vi "5 ch 2 samples minimum resonance scanner (FPGA) fixed pix clock.vi"() -> ()   [LabVIEW 2012]
uses:
  <vilib>/eio/EIONode/EIONode.xnode
  <vilib>/rvi/eio/common/nirviEmuTemplateMethod_errors.vi
  <vilib>/rvi/DataTransferAndStorage/Container/XNode/niFpgaContainer.xnode
  <vilib>/platform/TimedLoop/XDataNode/XDataNode.xnode
  <vilib>/Platform/TimedLoop/XDataNode/nitl_modes.ctl
  <vilib>/Platform/TimedLoop/XDataNode/XDNodeRunTimeDep.lvlib
  <vilib>/Platform/TimedLoop/XDataNode/wakeup.ctl
  <vilib>/Platform/TimedLoop/XDataNode/timing_clust.ctl
  <vilib>/rvi/interface/RandomDataEmulation/nirviRandomDataFpgaReadWriteTemplate.vi
panel:
  in  "lines at once":i16=4999
  in  "samples per half period":i16=4999
  in  "Start Delay (Ticks)":i16 caption="Start delay (Ticks)"
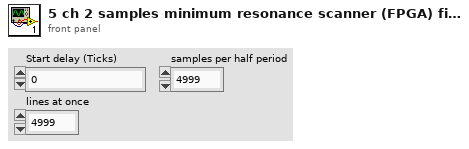
[diagram p1: front panel]
types:
  T1 = cluster{"IO Module\\AI A0":i16, "IO Module\\AI A1":i16, "IO Module\\AI A3":i16, "IO Module\\AI A6":i16}
  T2 = typedef "XDNodeRunTimeDep.lvlib/timing_clust.ctl" = cluster{"Expected End [f-1]":u64, "Actual End [f-1]":u64, "Finished Late? [f-1]":bool, "Expected End [i-1]":u64, "Actual End [i-1]":u64, "Finished Late? [i-1]":bool, "Expected Start [i]":u64, "Actual Start [i]":u64, "Expected Start [f]":u64, "Actual Start [f]":u64, "Source Name":string, "Structure Name":string, "Period":i64, "Deadline":i64, "Offset":i64, "Start":i64, "Priority":i32, "Timeout":i32, "Mode":T3, "Wakeup Reason":T4, "Error":errorcluster, "Source Type":string, "Secondary Source Type":string, "Global End Time":u64, "Global Start Time":u64, "Frame Duration":u64, "Iteration Duration":u64, "Assigned CPU":i32, "I/O Scan Engine Mode":u32}
  T3 = typedef "XDNodeRunTimeDep.lvlib/nitl_modes.ctl" = enum32{"No Change", "Process missed periods, maintain original phase", "Discard missed periods, maintain original phase", "Process missed periods, ignore original phase", "Discard missed periods, ignore original phase"}
  T4 = typedef "XDNodeRunTimeDep.lvlib/wakeup.ctl" = enum32{"Normal", "Aborted", "Asynchronous wakeup", "Timing source error", "Timed loop error", "Timeout"}
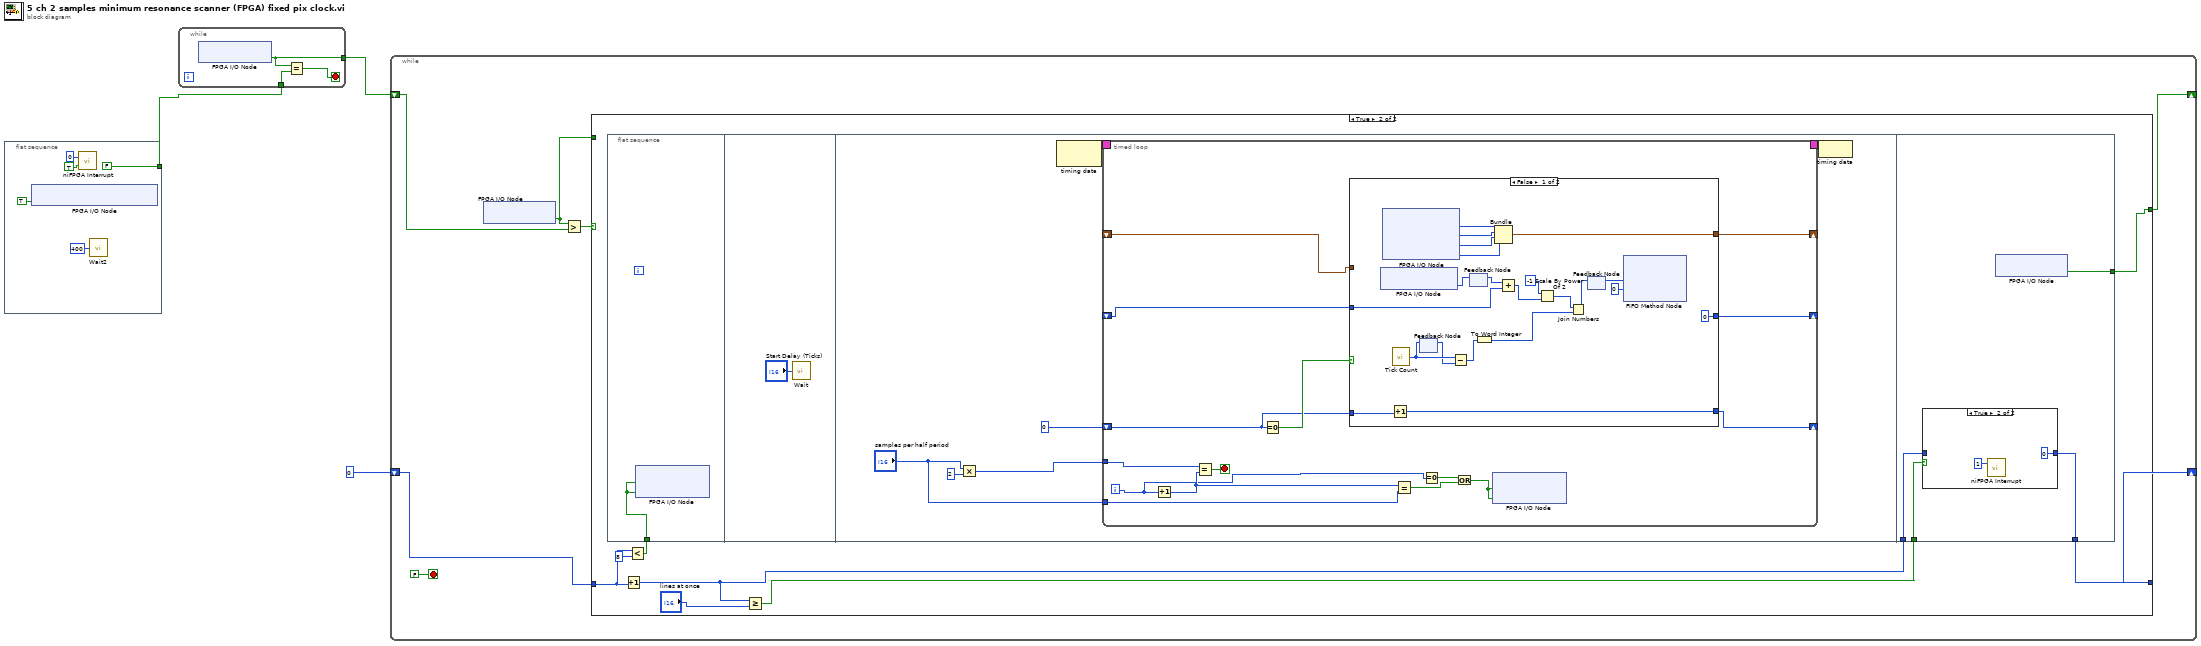
[diagram p0: block diagram]
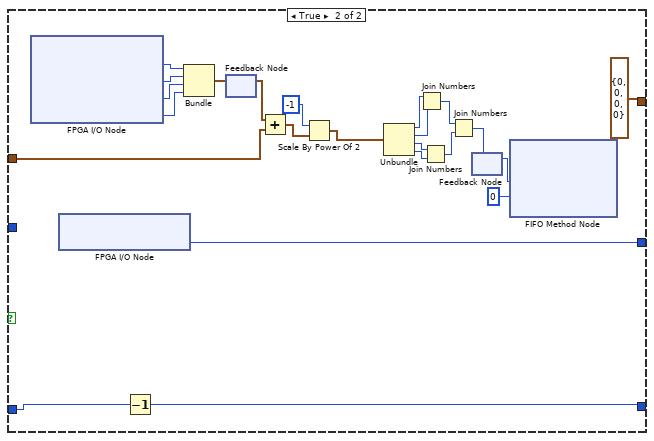
[diagram p3: hidden frame]
diagram:
  n1 = flat-sequence {
    tunnel: [FALSE ("IO Module\\DI 0")] -> w2
    frame #0 {
      n2 = xnode "FPGA I/O Node"("IO Module\\Digital Output Enable"=TRUE ("IO Module\\Digital Output Enable")) -> ()  [unwired: 1 in, 1 out]
      n3 = call <vilib>:"niFPGA Interrupt.vi"("Wait Until Cleared (F)"=TRUE, "IRQ Number (0)"=u8 0) -> ()  [unwired: 1 in]
      n4 = call "Wait2"("Count(mSec)"=u32 400) -> ()  [unwired: 1 out]
    }
  }
  n5 = while {
    tunnel: w2 -> [w11]
    tunnel: [w9] -> w1
    stop <- w10 stop-if-true
    n6 = xnode "FPGA I/O Node"() -> ("IO Module\\DI 0"=w9:bool)  [unwired: 1 in, 1 out]
    n7 = Equal?(x=w9, y=w11) -> (x = y?=w10:bool)
  }
  n8 = while {
    shift-right: [w17] -> _
    shift-left: w1 -> [w18]
    shift-right: [w15] -> _
    shift-left: i16 0 ("IRQ Number (0)") -> [w14]
    stop <- FALSE stop-if-true
    n9 = xnode "FPGA I/O Node"() -> ("IO Module\\DI 0"=w12:bool)  [unwired: 1 in, 1 out]
    n10 = Greater?(x=w12, y=w18) -> (0:w13:bool)
    n11 = case shown="True" w13 {
      tunnel: [w19 w21] -> w17
      tunnel: w14 -> [w20 w24]
      tunnel: [w20 w26] -> w15
      tunnel: w12 -> [w19 _]
      frame False {
      }
      frame True {
        n12 = flat-sequence {
          tunnel: w22 -> [w29]
          tunnel: w28 -> [w103]
          tunnel: w27 -> [w102]
          tunnel: [w101] -> w26
          tunnel: [w100] -> w21
          frame #0 {
            n13 = xnode "FPGA I/O Node"("PXI_Trig2"=w29, "IO Module\\D0 2"=w29) -> ()  [unwired: 2 in, 2 out]
          }
          frame #1 {
            n14 = call "Wait"("Count(Ticks)"="Start Delay (Ticks)") -> ()  [unwired: 1 out]
          }
          frame #2 {
            n15 = Multiply(x="samples per half period", y=i16 2) -> (x*y=w35:i16)
            n16 = node-c288() -> (w34:T2)  [unwired: 1 in]
            n17 = timed-loop {
              tunnel: w35 -> [w50]
              timing: w34 -> [_]
              timing-out: [_] -> w33
              shift-right: [w47] -> _
              shift-left: 0 ("Timeout") -> [w48]
              tunnel: "samples per half period" -> [w42]
              shift-right: [w40] -> _
              shift-left: _ -> [w39]
              shift-right: [w38] -> _
              shift-left: _ -> [w37]
              i -> [w41]
              stop <- w51 stop-if-true
              n18 = Increment(x=w41) -> (x+1=w43:i32)
              n19 = Equal?(x=w50, y=w43) -> (x = y?=w51:bool)
              n20 = Equal To 0?(x=w48) -> (x = 0?=w49:bool)
              n21 = case shown="False" w49 {
                tunnel: w48 -> [w72 w94]
                tunnel: [w71 w93] -> w47
                tunnel: [w61 T1 {"IO Module\\AI A0"=0, "IO Module\\AI A1"=0, "IO Module\\AI A3"=0, "IO Module\\AI A6"=0}] -> w40
                tunnel: w39 -> [_ w84]
                tunnel: [i16 0 ("IO Module\\AI B8") w77] -> w38
                tunnel: w37 -> [w58 _]
                frame False {
                  n22 = xnode "FPGA I/O Node"() -> ("IO Module\\AI B8"=w60:i16)  [unwired: 1 in, 1 out]
                  n23 = xnode "FPGA I/O Node"() -> ("IO Module\\AI A0"=w65:i16, "IO Module\\AI A1"=w64:i16, "IO Module\\AI A3"=w63:i16, "IO Module\\AI A6"=w62:i16)  [unwired: 4 in, 4 out]
                  n24 = Increment(x=w72) -> (x+1=w71:i32)
                  n25 = call "Tick Count"() -> ("Tick Count(Ticks)"=w70:u32)
                  n26 = feedback #1() -> (w69:u32)  [unwired: 1 in]
                  n27 = feedback-in #1(w70) -> ()
                  n28 = Subtract(x=w70, y=w69) -> (x-y=w68:u32)
                  n29 = feedback-in #2(w60) -> ()
                  n30 = feedback #2() -> (w59:i16)  [unwired: 1 in]
                  n31 = To Word Integer(number=w68) -> (16bit integer=w66:i16)
                  n32 = Bundle("IO Module\\AI A0"=w65, "IO Module\\AI A1"=w64, "IO Module\\AI A3"=w63, "IO Module\\AI A6"=w62) -> (w61:T1)  [unwired: 1 in]
                  n33 = Add(x=w59, y=w58) -> (x+y=w54:i16)
                  n34 = Scale By Power Of 2(n=i16 -1, x=w54) -> (x*2^n=w53:i16)
                  n35 = Join Numbers(hi=w53, lo=w66) -> ((hi.lo)=w57:u32)
                  n36 = feedback-in #3(w57) -> ()
                  n37 = feedback #3() -> (w52:u32)  [unwired: 1 in]
                  n38 = xnode ("FIFO Method Node")("Element"=w52, "Timeout"=0) -> ()  [unwired: 1 in, 2 out]
                }
                frame True {
                  n39 = xnode "FPGA I/O Node"() -> ("IO Module\\AI A0"=w90:i16, "IO Module\\AI A1"=w89:i16, "IO Module\\AI A3"=w88:i16, "IO Module\\AI A6"=w87:i16)  [unwired: 4 in, 4 out]
                  n40 = xnode "FPGA I/O Node"() -> ("IO Module\\AI B8"=w77:i16)  [unwired: 1 in, 1 out]
                  n41 = Decrement(x=w94) -> (x-1=w93:i32)
                  n42 = Bundle("IO Module\\AI A0"=w90, "IO Module\\AI A1"=w89, "IO Module\\AI A3"=w88, "IO Module\\AI A6"=w87) -> (w86:T1)  [unwired: 1 in]
                  n43 = feedback #4() -> (w85:T1)  [unwired: 1 in]
                  n44 = feedback-in #4(w86) -> ()
                  n45 = Add(x=w85, y=w84) -> (x+y=w76:T1)
                  n46 = Scale By Power Of 2(n=i16 -1, x=w76) -> (x*2^n=w74:T1)
                  n47 = Unbundle(w74) -> ("IO Module\\AI A0"=w83:i16, "IO Module\\AI A1"=w82:i16, "IO Module\\AI A3"=w81:i16, "IO Module\\AI A6"=w80:i16)
                  n48 = Join Numbers(hi=w83, lo=w82) -> ((hi.lo)=w91:u32)
                  n49 = Join Numbers(hi=w81, lo=w80) -> ((hi.lo)=w92:u32)
                  n50 = Join Numbers(hi=w91, lo=w92) -> ((hi.lo)=w79:u64)
                  n51 = feedback-in #5(w79) -> ()
                  n52 = feedback #5() -> (w73:u64)  [unwired: 1 in]
                  n53 = xnode ("FIFO Method Node")("Element"=w73, "Timeout"=0) -> ()  [unwired: 1 in, 2 out]
                }
              }
              n54 = Equal?(x=w43, y=w42) -> (x = y?=w45:bool)
              n55 = Equal To 0?(x=w41) -> (x = 0?=w46:bool)
              n56 = Or(x=w46, y=w45) -> (x .or. y?=w44:bool)
              n57 = xnode "FPGA I/O Node"("IO Module\\D0 1"=w44, "PXI_Trig1"=w44) -> ()  [unwired: 2 in, 2 out]
            }
            n58 = node-c288(w33) -> ()
          }
          frame #3 {
            n59 = case shown="True" w102 {
              tunnel: w103 -> [w104 _]
              tunnel: [w104 u8 0] -> w101
              frame False {
              }
              frame True {
                n60 = call <vilib>:"niFPGA Interrupt.vi"("IRQ Number (0)"=u8 1) -> ()  [unwired: 2 in]
              }
            }
            n61 = xnode "FPGA I/O Node"() -> ("IO Module\\DI 0"=w100:bool)  [unwired: 1 in, 1 out]
          }
        }
        n62 = Increment(x=w24) -> (x+1=w28:i16)
        n63 = Less?(x=w24, y=i16 8) -> (x < y?=w22:bool)
        n64 = Greater Or Equal?(x=w28, y="lines at once") -> (x >= y?=w27:bool)
      }
    }
  }
